vi "Actor Core.vi"(8 "error in":errorcluster, 11 "Nested in":refnum<class "Object Dictionary UI.lvclass">) -> (0 "error out":errorcluster, 3 "Actor out":refnum<class "Actor.lvclass">)   [LabVIEW 2024, in "Object Dictionary UI.lvlib" / "Object Dictionary UI.lvclass"]
doc: "(<B>Filename</B>: Actor Framework.lvlib:Actor.lvclass:Actor Core.vi)\n\nReceives messages to the actor, reacts to them, and initiates any error handling that may shut the actor down.\n\nDescendant classes may override this VI to append parallel tasks for the actor to complete while it handles messages. Overrides use the Call Parent Method node."
uses:
  Object Dictionary UI.lvclass
  <vilib>/ActorFramework/Actor/Actor.lvclass
  Object Dictionary UI.lvclass/Object Dictionary UI.ctl
  Object Dictionary UI Messages/Populate Entry Details Msg/Populate Entry Details Msg.lvclass
  Interactor Messages/Download OD Values Msg/Download OD Values Msg.lvclass
  Interactor Messages/Request OD Entry Values Msg/Request OD Entry Values Msg.lvclass
  <vilib>/ActorFramework/Stop Msg/Stop Msg.lvclass
  <vilib>/ActorFramework/Message Enqueuer/Message Enqueuer.lvclass
  <vilib>/MGI/Panel Manager/Panel Actor/Panel Actor/Panel Actor.lvclass
  C:/Program Files/National Instruments/LabVIEW 2025/vi.lib/MGI/Panel Manager/Panel Actor/Panel Actor/Panel Actor.lvclass
  C:/Program Files/National Instruments/LabVIEW 2025/vi.lib/ActorFramework/Actor/Actor.lvclass
  D:/git/CANopen-LabVIEW/Example/Object Dictionary UI/Object Dictionary UI.lvclass
  EDS-File-Viewer/source/Core/Electronic Datasheet.lvlib
  <vilib>/Utility/miscctls.llb/LVRowAndColumnUnsignedTypeDef.ctl
  <vilib>/MGI/Panel Manager/Panel/Panel Helper/Events.ctl
  <vilib>/MGI/Panel Manager/Panel/Panel Helper/Panel Helper.lvclass
  <vilib>/MGI/Panel Manager/Panel/Panel Helper/Panel Events.ctl
  EDS-File-Viewer/source/Core/Object Type.ctl
  EDS-File-Viewer/source/Core/Access SDO.ctl
  EDS-File-Viewer/source/Core/Access PDO.ctl
  EDS-File-Viewer/source/Core/Access SRDO.ctl
panel:
  out "Entry Details":T5 {"DataType" items=["UNKNOWN", "BOOLEAN", "INTEGER8", "INTEGER16", "INTEGER32", "UNSIGNED8", "UNSIGNED16", "UNSIGNED32", "REAL32", "VISIBLE_STRING", "OCTET_STRING", "UNICODE_STRING", "TIME_OF_DAY", "TIME_DIFFERENCE", "RESERVED1", "DOMAIN", "INTEGER24", "REAL64", "INTEGER40", "INTEGER48", "INTEGER56", "INTEGER64", "UNSIGNED24", "RESERVED2", "UNSIGNED40", "UNSIGNED48", "UNSIGNED56", "UNSIGNED64", "RESERVED3", "RESERVED4", "RESERVED5", "RESERVED6", "PDO_COMMUNICATION_PARAMETER", "PDO_MAPPING", "SDO_PARAMETER", "IDENTITY", "RESERVED7"]; "ObjectType" items=["NULL"=0, "DOMAIN"=2, "DEFTYPE"=5, "DEFSTRUCT"=6, "VAR"=7, "ARRAY"=8, "RECORD"=9]}
  in  "Attribute Table":string[][](table)
  out "Device Profile Specific":string[][](table)
  out "Manufacturer Specific":string[][](table)
  out "Communication Specific":string[][](table)
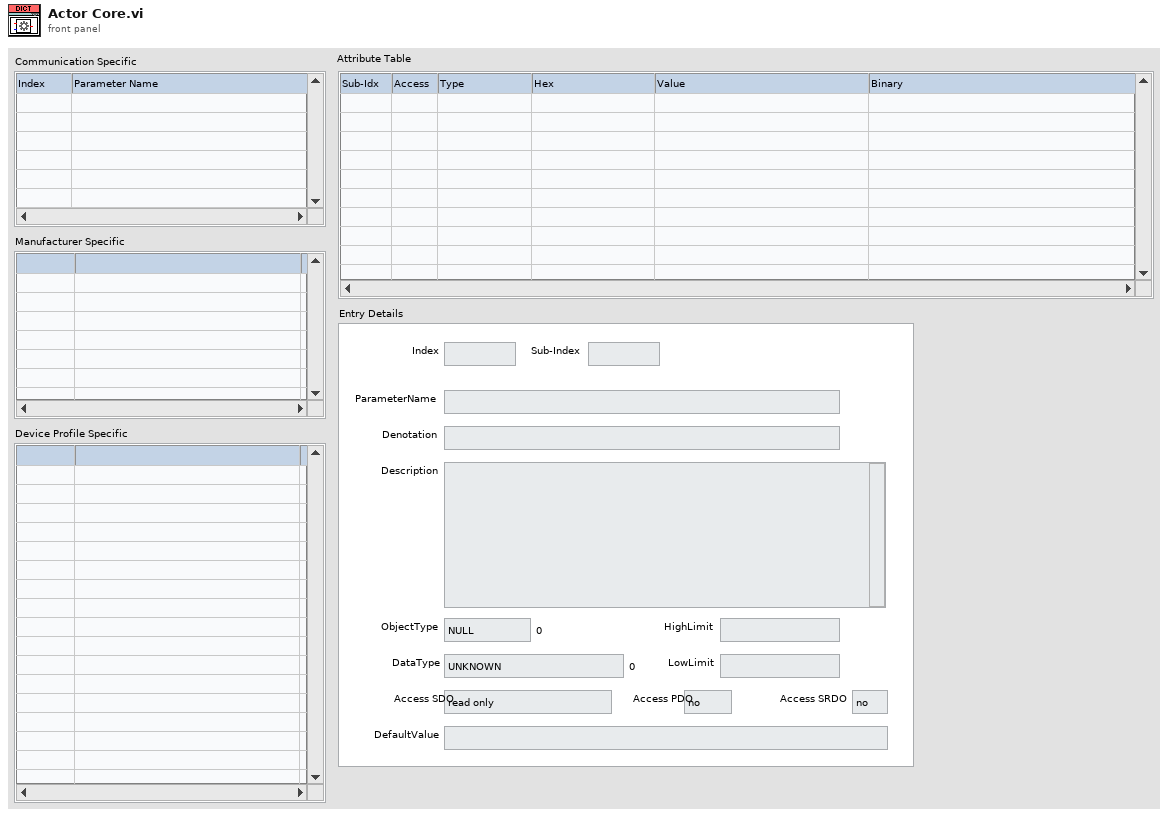
[diagram p1: front panel]
types:
  T1 = typedef "Electronic Datasheet.lvlib/Object Type.ctl" = u8
  T2 = typedef "Electronic Datasheet.lvlib/Access SDO.ctl" = enum16{"read only", "write only", "read/write", "read/write on process input", "read/write on process output", "constant value", "no", "UNKNOWN"}
  T3 = typedef "Electronic Datasheet.lvlib/Access PDO.ctl" = enum16{"no", "TPDO", "RPDO", "TPDO & RPDO"}
  T4 = typedef "Electronic Datasheet.lvlib/Access SRDO.ctl" = enum16{"no", "tx", "rx", "trx"}
  T5 = cluster{"Index":string, "Sub-Index":string, "ParameterName":string, "Denotation":string, "Description":string, "ObjectType":T1, "HighLimit":string, "DataType":u16, "LowLimit":string, "Access SDO":T2, "Access PDO":T3, "Access SRDO":T4, "DefaultValue":string}
  T6 = cluster{"Pnl Actor":refnum<event-registration>, "Custom":refnum<event-registration>}
  T7 = typedef "LVRowAndColumnUnsignedTypeDef.ctl" = cluster{"Row":u32, "Column":u32}
  T8 = enum8{"Enabled", "Disabled", "Disabled and Grayed Out"}
  T9 = cluster{"Communication Specific Objects":refnum<user-event>, "Attribute Table":refnum<user-event>, "Entry Details":refnum<user-event>}
  T10 = cluster{"Multiplexer":cluster{"Index":u16, "Sub-Index":i16}, "Value":variant}
  T11 = typedef "LVPoint32TypeDef.ctl" = cluster{"Horizontal":i32, "Vertical":i32}
  T12 = typedef "LVRowAndColumnTypeDef.ctl" = cluster{"Row":i32, "Column":i32}
  T13 = cluster{"Multiplexer":cluster{"Index":u16, "Sub-Index":i16}, "Value":variant}[]
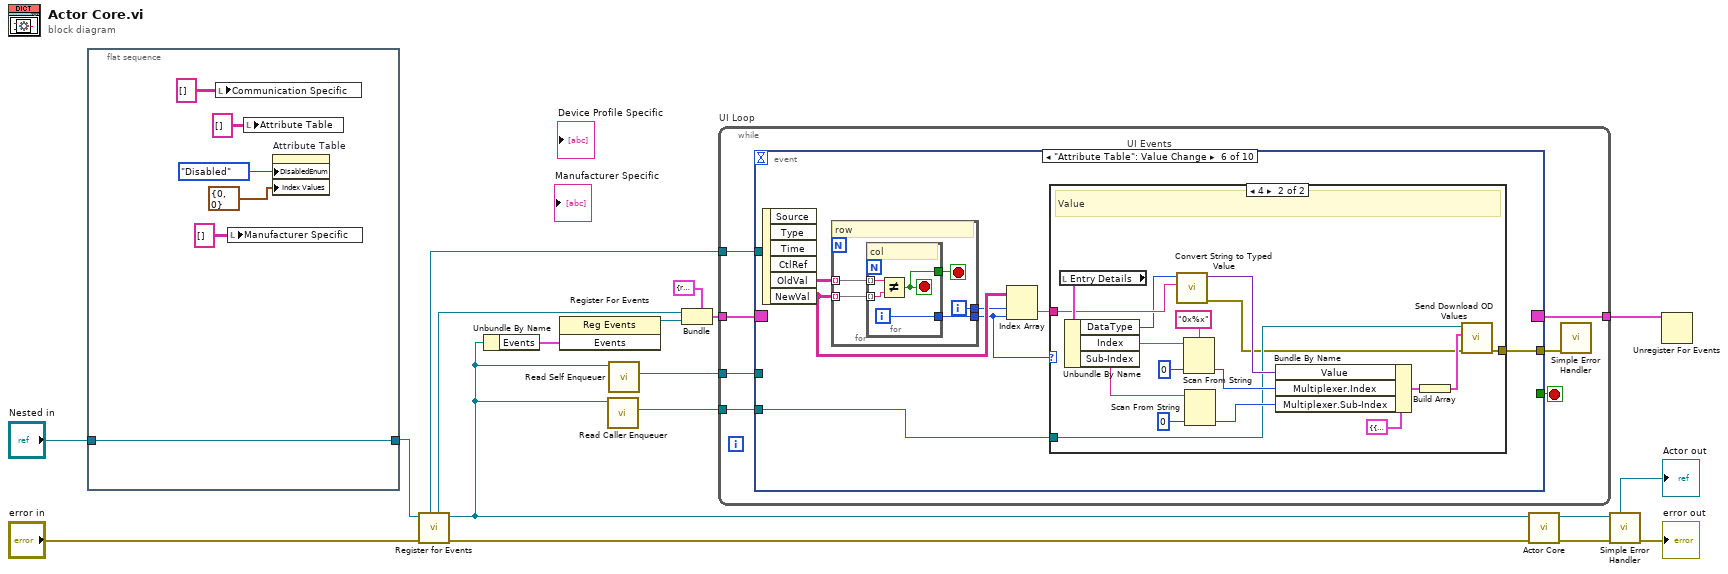
[diagram p0: block diagram]
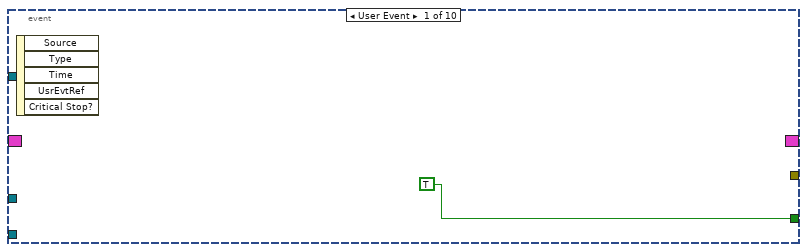
[diagram p2: hidden frame]
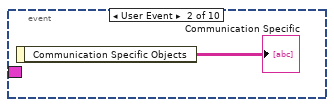
[diagram p3: hidden frame]
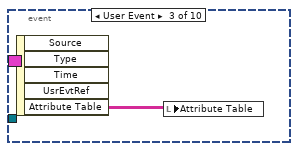
[diagram p4: hidden frame]
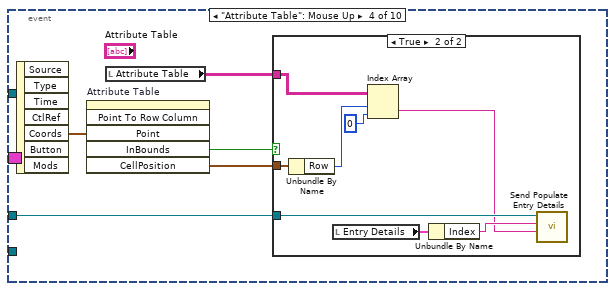
[diagram p5: hidden frame]
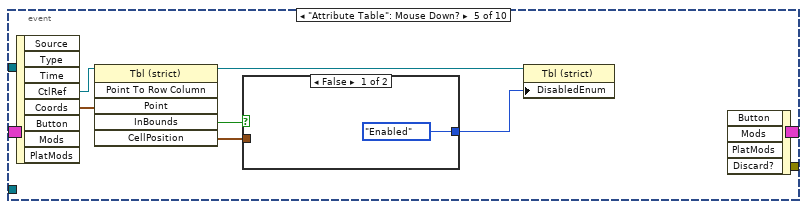
[diagram p7: hidden frame]
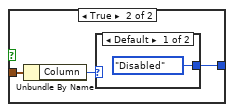
[diagram p8: hidden frame]
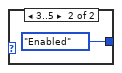
[diagram p9: hidden frame]
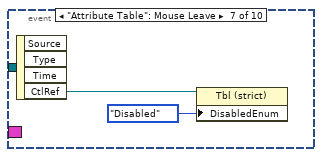
[diagram p11: hidden frame]
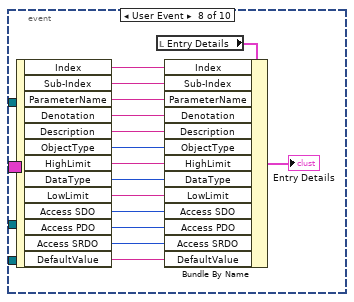
[diagram p12: hidden frame]
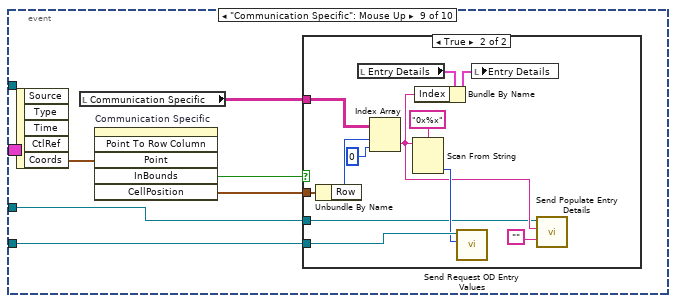
[diagram p13: hidden frame]
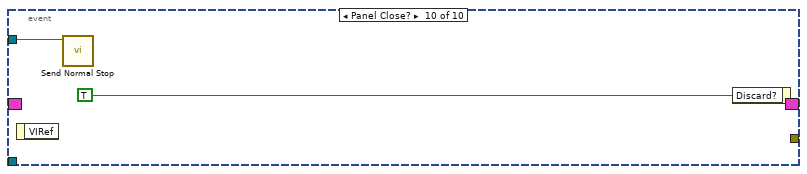
[diagram p15: hidden frame]
diagram:
  n1 = flat-sequence {
    tunnel: "Nested in" -> [w23]
    tunnel: [w23] -> w7
    frame #0 {
      n2 = local write "Communication Specific"(string[][] [] ("Communication Specific")) -> ()
      n3 = local write "Manufacturer Specific"(string[][] [] ("Manufacturer Specific")) -> ()
      n4 = local write "Attribute Table"(string[][] [] ("Attribute Table")) -> ()
      n5 = property on="Attribute Table" class="Tbl (strict)"("DisabledEnum"=T8."Disabled" ("Disabled"), "Index Values"=T7 {"Row"=0, "Column"=0}) -> ()  [unwired: 2 in, 2 out]
    }
  }
  n6 = call <vilib>:"Register for Events.vi"("Error In"="error in", "Panel Actor in"=w7) -> ("Error Out"=w9:errorcluster, "Panel Actor out"=w3:refnum<class "Object Dictionary UI.lvclass">, "Pnl Actor"=w10:refnum<event-registration>, "Self Enqueuer"=w12:refnum<class "Message Enqueuer.lvclass">)  [unwired: 6 in]
  n7 = Unbundle By Name(w3) -> ("Events"=w15:T9)
  n8 = register-events ("Main Register for Events")(w15) -> (reference out=w5:refnum<event-registration>)  [unwired: 2 in, 1 out]
  n9 = call <vilib>:"Read Caller Enqueuer.vi"("Actor"=w3) -> ("Caller Enqueuer"=w6:refnum<class "Message Enqueuer.lvclass">)  [unwired: 10 in]
  n10 = call <vilib>:"Read Self Enqueuer.vi"("Actor"=w3) -> ("Self Enqueuer"=w2:refnum<class "Message Enqueuer.lvclass">)  [unwired: 10 in]
  n11 = Bundle(cluster=T6 {"Pnl Actor"=refnum, "Custom"=refnum}, "Pnl Actor"=w10, "Custom"=w5) -> (w11:T6)
  n12 = while "UI Loop" {
    tunnel: w11 -> [w30]
    tunnel: [w28] -> w14
    tunnel: w12 -> [w27]
    tunnel: w6 -> [w26]
    tunnel: w2 -> [w25]
    stop <- w29 stop-if-true
    n13 = event "UI Events" shown="[5] \"Attribute Table\": Value Change" {
      selector: w30 -> [_ _ _ _ _ _ _ _ _ _]
      dyn-events: [_ _ _ _ _ _ _ _ _ _] -> w28
      timeout: _ -> [_ _ _ _ _ _ _ _ _ _]
      tunnel: [TRUE _ _ _ _ _ _ _ _ _] -> w29
      tunnel: w27 -> [_ _ _ _ _ _ _ _ _ w127]
      tunnel: w26 -> [_ _ _ _ _ w59 _ _ w111 _]
      tunnel: w25 -> [_ _ _ w34 _ _ _ _ w109 _]
      tunnel: [_ _ _ _ _ w60 _ _ _ _] -> w24
      event User Event {
        n14 = event-data() -> ()  [unwired: 1 in, 5 out]
      }
      event User Event {
        n15 = event-data() -> ("Communication Specific Objects"=→"Communication Specific":string[][])  [unwired: 1 in]
      }
      event User Event {
        n16 = event-data() -> ("Attribute Table"=w33:string[][])  [unwired: 1 in, 4 out]
        n17 = local write "Attribute Table"(w33) -> ()
      }
      event "Attribute Table": Mouse Up {
        n18 = event-data() -> ("Coords"=w38:T11)  [unwired: 1 in, 6 out]
        n19 = invoke on="Attribute Table" class="Tbl (strict)" method="Point To Row Column"("Point"=w38) -> ("InBounds"=w37:bool, "CellPosition"=w36:T12)  [unwired: 5 in, 4 out]
        n20 = local read "Attribute Table"() -> (w35:string[][])
        n21 = case shown="True" w37 {
          tunnel: w36 -> [_ w46]
          tunnel: w35 -> [_ w44]
          tunnel: w34 -> [_ w42]
          frame False {
          }
          frame True {
            n22 = Unbundle By Name(w46) -> ("Row"=w43:i32)
            n23 = local read "Entry Details"() -> (w41:T5)
            n24 = Index Array(array=w44, index (row)=w43, index (col)=0) -> (element=w39:string)
            n25 = Unbundle By Name(w41) -> ("Index"=w40:string)
            n26 = call "Send Populate Entry Details.vi"("Sub-Index"=w39, "Index"=w40, "Message Enqueuer"=w42) -> ()  [unwired: 7 in, 2 out]
          }
        }
      }
      event "Attribute Table": Mouse Down? {
        n27 = event-data() -> ("CtlRef"=w48:refnum<vi>, "Coords"=w49:T11)  [unwired: 1 in, 6 out]
        n28 = invoke class="Tbl (strict)" method="Point To Row Column"(reference=w48, "Point"=w49) -> (reference out=w50:refnum<vi>, "InBounds"=w52:bool, "CellPosition"=w51:T12)  [unwired: 4 in, 3 out]
        n29 = case shown="False" w52 {
          tunnel: w51 -> [_ w56]
          tunnel: [T8."Enabled" ("Disabled") w54] -> w47
          frame False {
          }
          frame True {
            n30 = Unbundle By Name(w56) -> ("Column"=w55:i32)
            n31 = case shown="Default" w55 {
              tunnel: [T8."Disabled" ("Disabled") T8."Enabled" ("Disabled")] -> w54
              frame Default {
              }
              frame 3..5 {
              }
            }
          }
        }
        n32 = property class="Tbl (strict)"(reference=w50, "DisabledEnum"=w47) -> ()  [unwired: 1 in, 2 out]
        n33 = event-data() -> ()  [unwired: 5 in, 1 out]
      }
      event "Attribute Table": Value Change {
        n34 = event-data() -> ("OldVal"=w65:string[][], "NewVal"=w64:string[][])  [unwired: 1 in, 4 out]
        n35 = for {
          tunnel: w65 -> [w70] mode=indexing
          tunnel: w64 -> [w69] mode=indexing
          tunnel: [w68] -> w62
          tunnel: [w67] -> w63
          i -> [w67]
          stop <- w66 stop-if-true
          # "row"
          n36 = for {
            tunnel: w70 -> [w74] mode=indexing
            tunnel: w69 -> [w73] mode=indexing
            tunnel: [w72] -> w68
            tunnel: [w71] -> w66
            i -> [w72]
            stop <- w71 stop-if-true
            # "col"
            n37 = Not Equal?(x=w74, y=w73) -> (x != y?=w71:bool)
          }
        }
        n38 = Index Array(array=w64, index (row)=w63, index (col)=w62) -> (element=w61:string)
        n39 = case shown="4" w62 {
          tunnel: w61 -> [_ w90]
          tunnel: [_ w76] -> w60
          tunnel: w59 -> [_ w78]
          frame 0, Default {
          }
          frame 4 {
            # "Value"
            n40 = local read "Entry Details"() -> (w91:T5)
            n41 = Unbundle By Name(w91) -> ("DataType"=w89:u16, "Index"=w84:string, "Sub-Index"=w79:string)
            n42 = call "Convert String to Typed Value.vi"("Value"=w90, "DataType"=w89) -> ("error out"=w77:errorcluster, "Typed Value"=w87:variant)  [unwired: 8 in]
            n43 = Scan From String(format string="0x%x", input string=w84, default 1=u16 0 ("Multiplexer.Index")) -> (output 1=w83:u16)  [unwired: 2 in, 3 out]
            n44 = Scan From String(input string=w79, default 1=i16 0 ("Multiplexer.Sub-Index")) -> (output 1=w80:i16)  [unwired: 3 in, 3 out]
            n45 = Bundle By Name(cluster=T10 {"Multiplexer"={"Index"=0, "Sub-Index"=0}, "Value"=variant}, "Value"=w87, "Multiplexer.Index"=w83, "Multiplexer.Sub-Index"=w80) -> (w85:T10)
            n46 = Build Array(w85) -> (w86:T13)
            n47 = call "Send Download OD Values.vi"("error in (no error)"=w77, "Values"=w86, "Message Enqueuer"=w78) -> ("error out"=w76:errorcluster)  [unwired: 7 in, 1 out]
          }
        }
      }
      event "Attribute Table": Mouse Leave {
        n48 = event-data() -> ("CtlRef"=w93:refnum<vi>)  [unwired: 1 in, 3 out]
        n49 = property class="Tbl (strict)"(reference=w93, "DisabledEnum"=T8."Disabled" ("Disabled")) -> ()  [unwired: 1 in, 2 out]
      }
      event User Event {
        n50 = event-data() -> ("Index"=w107:string, "Sub-Index"=w106:string, "ParameterName"=w105:string, "Denotation"=w104:string, "Description"=w103:string, "ObjectType"=w102:T1, "HighLimit"=w101:string, "DataType"=w100:u16, "LowLimit"=w99:string, "Access SDO"=w98:T2, "Access PDO"=w97:T3, "Access SRDO"=w96:T4, "DefaultValue"=w95:string)  [unwired: 1 in]
        n51 = local read "Entry Details"() -> (w108:T5)
        n52 = Bundle By Name(cluster=w108, "Index"=w107, "Sub-Index"=w106, "ParameterName"=w105, "Denotation"=w104, "Description"=w103, "ObjectType"=w102, "HighLimit"=w101, "DataType"=w100, "LowLimit"=w99, "Access SDO"=w98, "Access PDO"=w97, "Access SRDO"=w96, "DefaultValue"=w95) -> (→"Entry Details":T5)
      }
      event "Communication Specific": Mouse Up {
        n53 = event-data() -> ("Coords"=w114:T11)  [unwired: 1 in, 4 out]
        n54 = local read "Communication Specific"() -> (w112:string[][])
        n55 = invoke on="Communication Specific" class="Tbl (strict)" method="Point To Row Column"("Point"=w114) -> ("InBounds"=w110:bool, "CellPosition"=w113:T12)  [unwired: 5 in, 4 out]
        n56 = case shown="True" w110 {
          tunnel: w113 -> [_ w126]
          tunnel: w112 -> [_ w125]
          tunnel: w111 -> [_ w121]
          tunnel: w109 -> [_ w115]
          frame False {
          }
          frame True {
            n57 = Unbundle By Name(w126) -> ("Row"=w124:i32)
            n58 = local read "Entry Details"() -> (w119:T5)
            n59 = Index Array(array=w125, index (row)=w124, index (col)=0) -> (element=w117:string)
            n60 = Scan From String(format string="0x%x", input string=w117) -> (output 1=w120:u16)  [unwired: 3 in, 3 out]
            n61 = Bundle By Name(cluster=w119, "Index"=w117) -> (w118:T5)
            n62 = call "Send Request OD Entry Values.vi"("Index"=w120, "Message Enqueuer"=w121) -> ()  [unwired: 8 in, 2 out]
            n63 = local write "Entry Details"(w118) -> ()
            n64 = call "Send Populate Entry Details.vi"("Sub-Index"="", "Index"=w117, "Message Enqueuer"=w115) -> ()  [unwired: 7 in, 2 out]
          }
        }
      }
      event Panel Close? {
        n65 = event-data() -> ()  [unwired: 1 in, 1 out]
        n66 = call <vilib>:"Send Normal Stop.vi"("Message Enqueuer"=w127) -> ()  [unwired: 10 in, 1 out]
        n67 = event-data("Discard?"=TRUE) -> ()  [unwired: 1 in, 1 out]
      }
    }
    n68 = call <vilib>:"Simple Error Handler.vi"("error in (no error)"=w24) -> ()  [unwired: 4 in, 5 out]
  }
  n69 = call-parent "Actor Core.vi"("error in"=w9, "Panel Actor in"=w3) -> ("error out"=w17:errorcluster, "Actor out"=→"Actor out":refnum<class "Actor.lvclass">)  [unwired: 8 in]
  n70 = call <vilib>:"Simple Error Handler.vi"("error in (no error)"=w17) -> ("error out"=→"error out":errorcluster)  [unwired: 4 in, 4 out]
  n71 = Unregister For Events(event registration refnum=w14) -> ()  [unwired: 1 in, 1 out]
